vi "add channel.vi"(7 "owner ID":string, 8 "error in":errorcluster, 10 "channel descriptor":refnum<class "TBM channel.lvclass">, 11 "engine configuration in":refnum<class "base TBM sequencer configuration.lvclass">) -> (0 "error out":errorcluster, 3 "engine configuration out":refnum<class "base TBM sequencer configuration.lvclass">)   [LabVIEW 2014, in "base TBM sequencer configuration.lvclass"]
uses:
  base TBM sequencer configuration.lvclass
  <vilib>/NI/Tag Bus Module Framework/channel/TBM channel.lvclass
  <vilib>/NI/Tag Bus/tag/tag descriptor.lvclass/tag descriptor.ctl
  Tag Info.ctl
  base TBM sequencer configuration.lvclass/base TBM sequencer configuration.ctl
  <vilib>/NI/Tag Bus/tag/read tag name.vi
  <vilib>/NI/Configuration Framework/NISE_CEF_TreeControl.lvlib
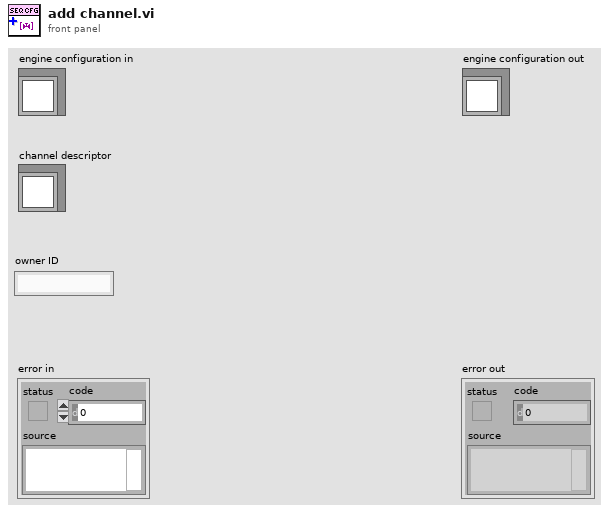
[diagram p1: front panel]
types:
  T1 = typedef "base TBM sequencer configuration.lvclass/Tag Info.ctl" = cluster{"Channel":refnum<class "TBM channel.lvclass">, "Writers":string[], "Readers":string[], "Owning ID":string}
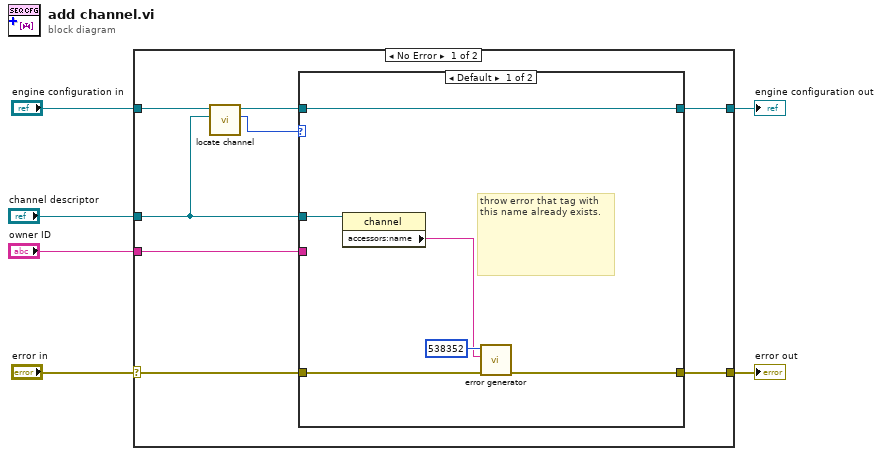
[diagram p0: block diagram]
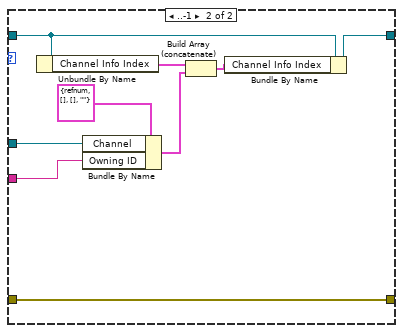
[diagram p2: hidden frame]
diagram:
  n1 = case shown="No Error" "error in" {
    selector: "error in" -> [w10 w31]
    tunnel: [w9 w31] -> w5
    tunnel: [w11 w30] -> w3
    tunnel: "engine configuration in" -> [w14 w30]
    tunnel: "channel descriptor" -> [w8 _]
    tunnel: "owner ID" -> [w7 _]
    frame No Error {
      n2 = call "locate channel.vi"("tag descriptor"=w8, "sequencer config in"=w14) -> ("index"=w13:i32, "sequencer config out"=w12:refnum<class "base TBM sequencer configuration.lvclass">)  [unwired: 8 in]
      n3 = case shown="Default" w13 {
        tunnel: w12 -> [w20 w24]
        tunnel: [w20 w22] -> w11
        tunnel: w10 -> [w18 w29]
        tunnel: [w17 w29] -> w9
        tunnel: w8 -> [w16 w26]
        tunnel: w7 -> [_ w21]
        frame Default {
          # "throw error that tag with this name already exists."
          n4 = property class="channel"(reference=w16) -> ("accessors:name"=w15:string)  [unwired: 1 in, 2 out]
          n5 = call <vilib>:"error generator.vi"("error in"=w18, "append error message"=w15, "error code (0)"=538352) -> ("error out"=w17:errorcluster)  [unwired: 6 in]
        }
        frame ..-1 {
          n6 = Unbundle By Name(w24) -> ("Channel Info Index"=w28:T1[])
          n7 = Bundle By Name(cluster=T1 {"Channel"=refnum, "Writers"=[], "Readers"=[], "Owning ID"=""} ("Tag Info"), "Channel"=w26, "Owning ID"=w21) -> (w25:T1)
          n8 = Build Array (concatenate)(w28, w25) -> (w23:T1[])
          n9 = Bundle By Name(cluster=w24, "Channel Info Index"=w23) -> (w22:refnum<class "base TBM sequencer configuration.lvclass">)
        }
      }
    }
    frame Error {
    }
  }
  "error out" <- w5
  "engine configuration out" <- w3
